vi "FileIO_MoveFile.vi"(0 "Source Path":path, 5 "Target Path":path, 11 "Error In":errorcluster) -> (4 "New Path":path, 15 "Error Out":errorcluster)   [LabVIEW 2016]
doc: "This VI will move a file from one directory to another. It does not copy the file, therefore file will only be in new location."
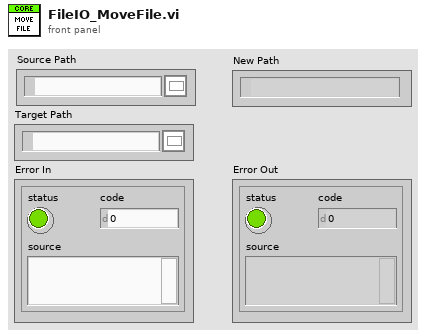
[diagram p1: front panel]
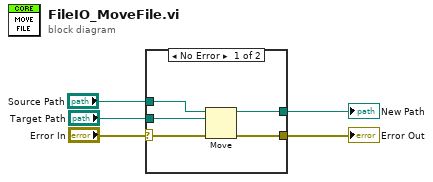
[diagram p0: block diagram]
diagram:
  n1 = case shown="No Error" "Error In" {
    selector: "Error In" -> [w10 w11]
    tunnel: "Target Path" -> [w8 _]
    tunnel: [w9 w11] -> w4
    tunnel: "Source Path" -> [w7 _]
    tunnel: [w6 _] -> w1
    frame No Error {
      n2 = Move(source path=w7, error in=w10, 10:w8) -> (error out=w9:errorcluster, 3:w6:path)  [unwired: 2 in, 1 out]
    }
    frame Error {
    }
  }
  "Error Out" <- w4
  "New Path" <- w1
